vi "Add Chart Area.vi"(8 "error in (no error)":errorcluster, 10 ".NET MSChart ChartArea":refnum<k24>, 11 ".NET MSChart":refnum<k24>) -> (0 "error out":errorcluster)   [LabVIEW 2015, in "Graph Extensions MSChart.lvlib"]
uses:
  Graph Extensions MSChart.lvlib
  System.Windows.Forms.DataVisualization
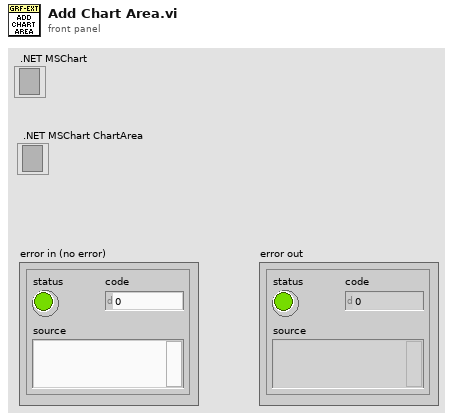
[diagram p1: front panel]
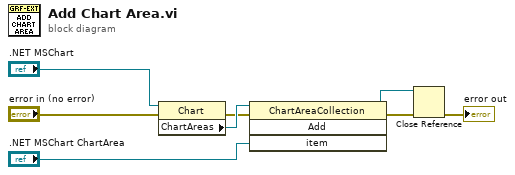
[diagram p0: block diagram]
diagram:
  n1 = property class="Chart"(reference=".NET MSChart", error in="error in (no error)") -> (error out=w5:errorcluster, "ChartAreas"=w6:refnum<k24>)  [unwired: 1 out]
  n2 = invoke class="ChartAreaCollection" method="Add"(reference=w6, error in=w5, "item"=".NET MSChart ChartArea") -> (reference out=w4:refnum<k24>, error out=w3:errorcluster)  [unwired: 1 in, 2 out]
  n3 = Close Reference(reference=w4, error in (no error)=w3) -> (error out=→"error out":errorcluster)
